vi "EditParam.vi"(10 "type":u16(ring)=2 items=["USB-CAN"=2, "USB-CAN2.0"=3], 11 "param":T1[](array[typedef]) {"ACR0" format="%x"}) -> (3 "param out":T1[](array[typedef]) {"ACR0" format="%x"})   [LabVIEW 2011]
uses:
  Param.ctl
panel:
  in  "m2":enum16{"ANY", "IDE"}(ring) caption="过滤模式:"
  in  "m1":enum16{"标准帧", "扩展帧"}(ring) caption="过滤模式:"
  in  "m0":enum16{"标准帧", "扩展帧"}(ring) caption="过滤模式组合:"
  in  "Cancel":bool
  in  "OK":bool
  in  "channel":enum16{"通道1", "通道2"}(ring) caption="选择要编辑的CAN通道号："
  in  "屏蔽码":u32=4294967295 caption="屏蔽码:" format="0x%08x"
  in  "验收码":u32=2147483648 caption="验收码:" format="0x%08x"
  in  "工作模式:":u16(ring) items=["正常工作", "自测模试（环回模式）", "仅监帧听模式", "监听所有信息模式", "关闭模式", "配置模式"]
  in  "BTR1":u8=28 caption="(HEX)" format="%02x"
  in  "BTR0":u8=1 caption="BTR0/1:" format="%02x"
  in  "br":u32(ring)=8 caption="波特率:" items=["5k bps"=1, "10k bps"=2, "20k bps"=3, "40k bps"=4, "50k bps"=5, "80k bps"=6, "100k bps"=7, "125k bps"=8, "200k bps"=9, "250k bps"=10, "400k bps"=11, "500k bps"=12, "666k bps"=13, "800k bps"=14, "1000k bps"=15, "self define"=16]
  # "CAN初始化参数"
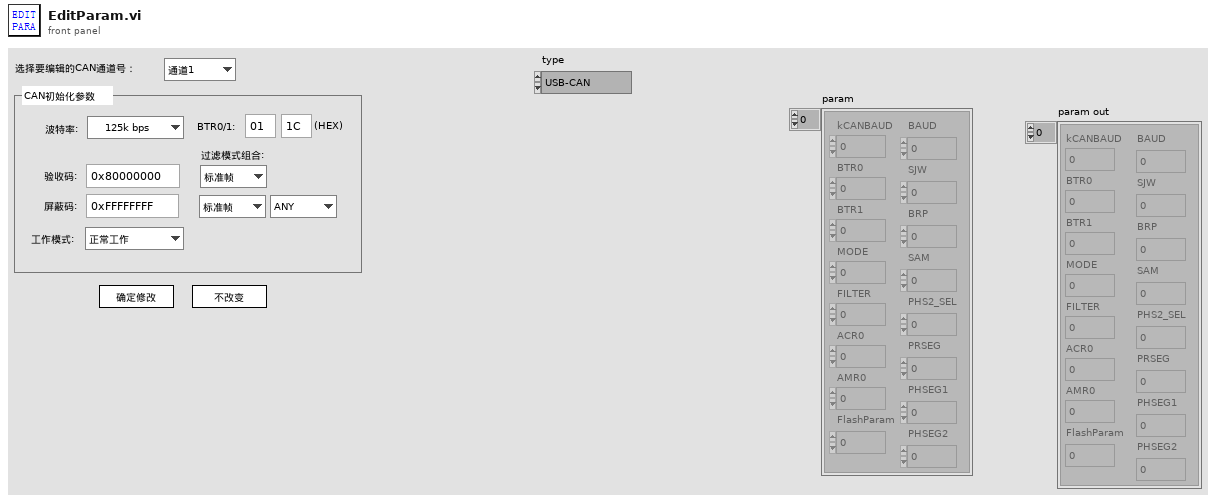
[diagram p1: front panel]
types:
  T1 = typedef "Param.ctl" = cluster{"kCANBAUD":u8, "BTR0":u8, "BTR1":u8, "MODE":u8, "FILTER":u8, "ACR0":u32, "AMR0":u32, "FlashParam":u32, "BAUD":u32, "SJW":u8, "BRP":u8, "SAM":u8, "PHS2_SEL":u8, "PRSEG":u8, "PHSEG1":u8, "PHSEG2":u8}
  T2 = enum8{"Enabled", "Disabled", "Disabled and Grayed Out"}
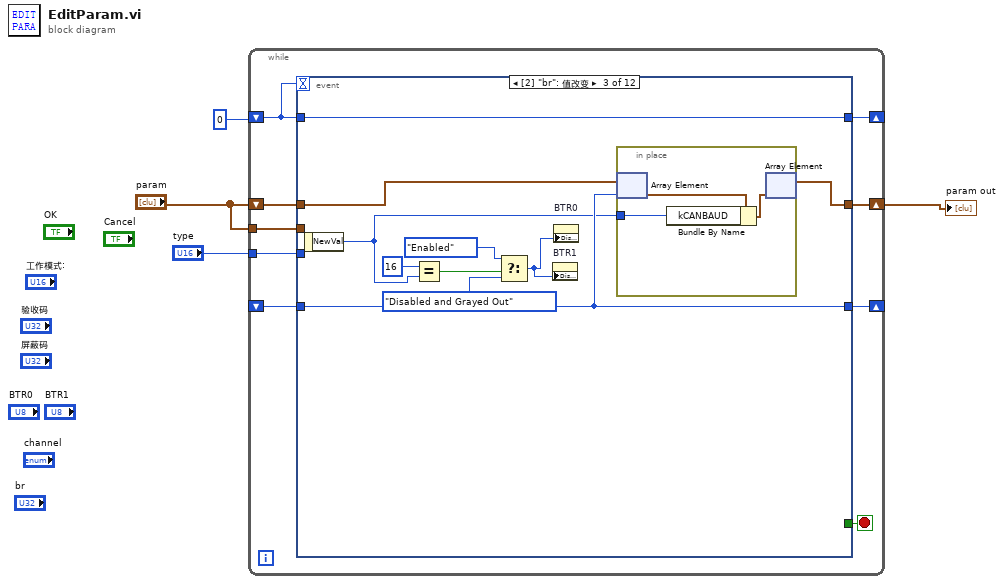
[diagram p0: block diagram]
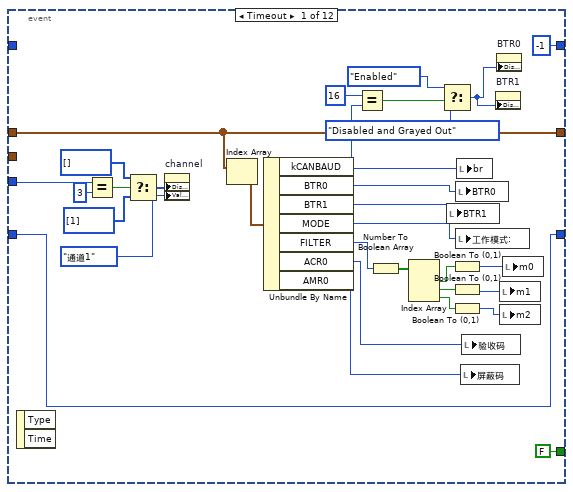
[diagram p2: hidden frame]
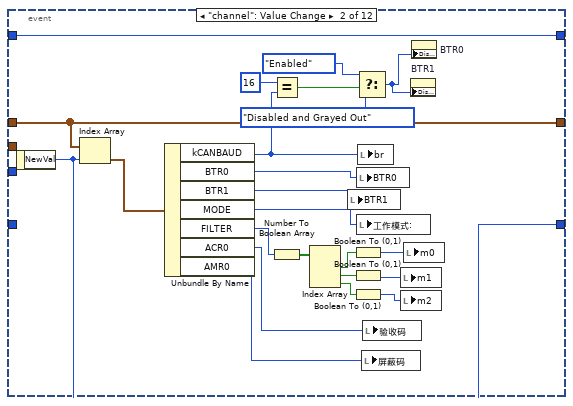
[diagram p3: hidden frame]
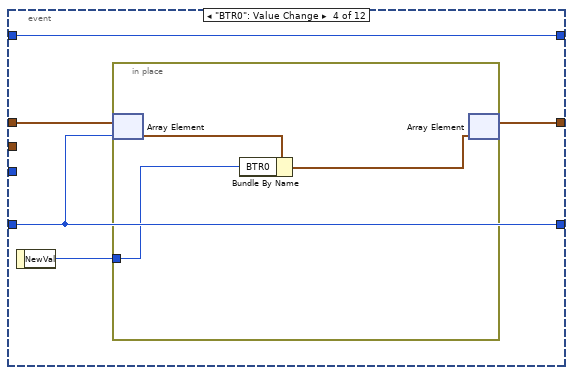
[diagram p4: hidden frame]
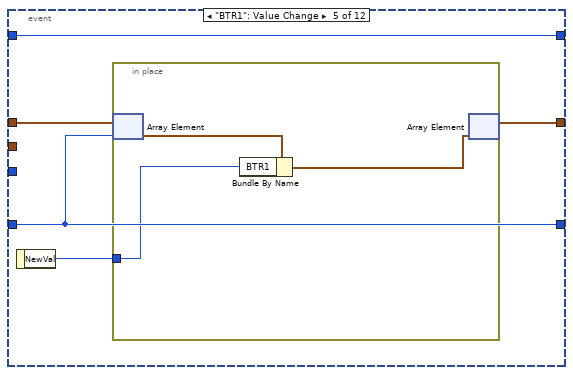
[diagram p5: hidden frame]
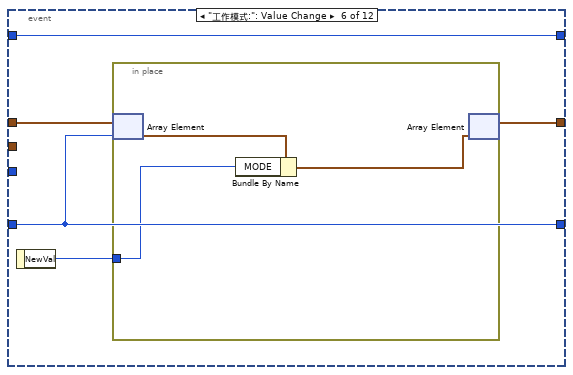
[diagram p6: hidden frame]
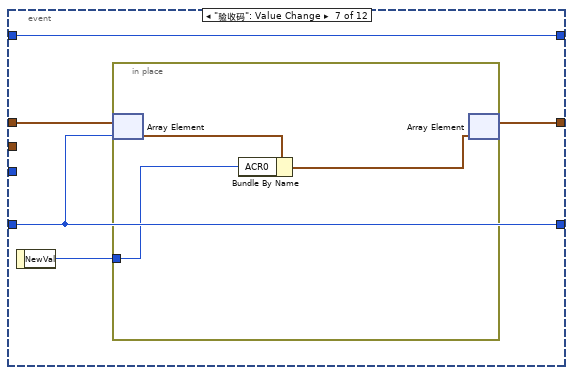
[diagram p7: hidden frame]
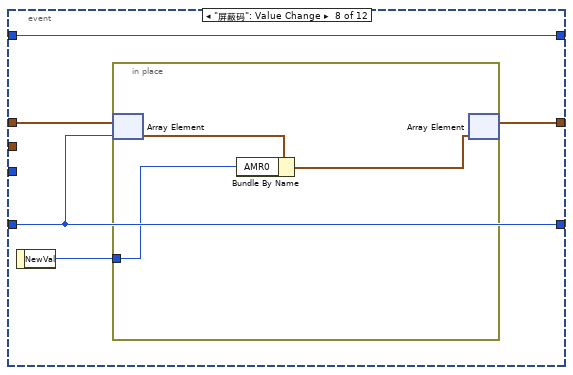
[diagram p8: hidden frame]
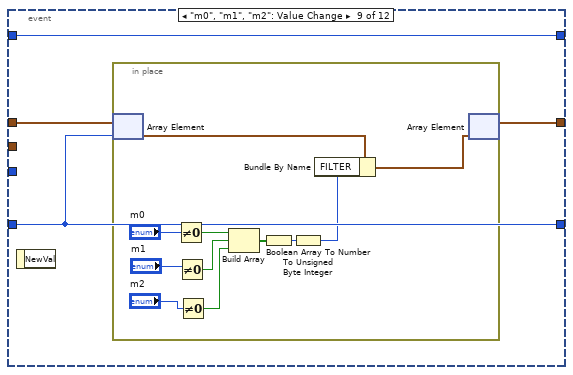
[diagram p9: hidden frame]
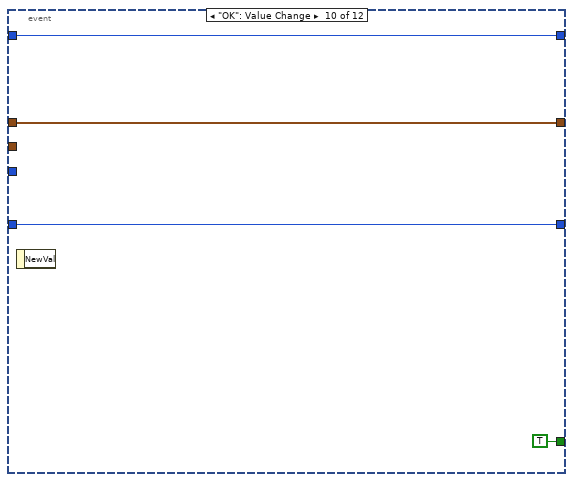
[diagram p10: hidden frame]
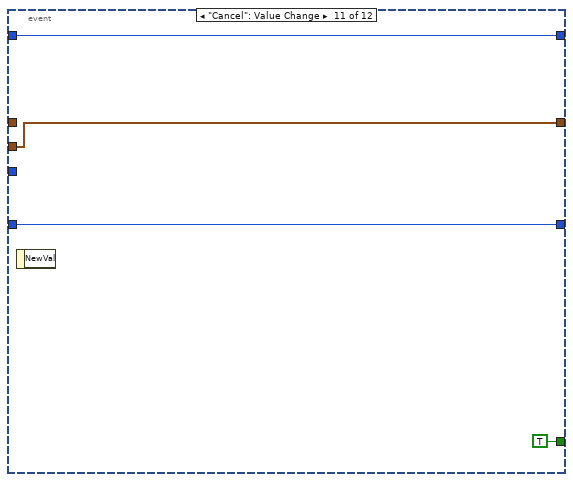
[diagram p11: hidden frame]
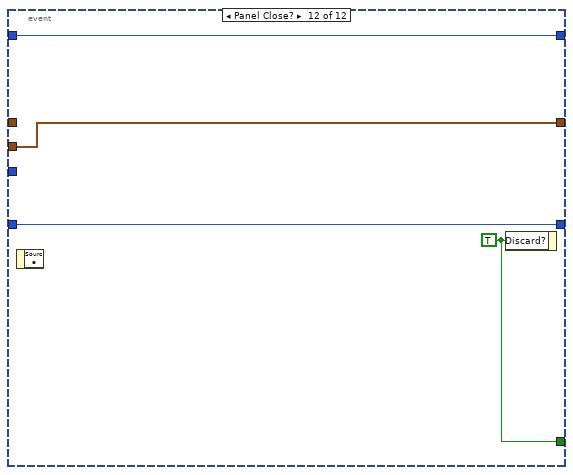
[diagram p12: hidden frame]
diagram:
  n1 = while {
    shift-right: [w11] -> w2
    shift-left: "param" -> [w12]
    shift-right: [w10] -> _
    shift-left: 0 -> [w9]
    tunnel: "type" -> [w8]
    shift-right: [w7] -> _
    shift-left: _ -> [w6]
    tunnel: "param" -> [w5]
    stop <- w13 stop-if-true
    n2 = event shown="[2] \"br\": 值改变" {
      selector: _ -> [_ _ _ _ _ _ _ _ _ _ _ _]
      dyn-events: _ -> [_ _ _ _ _ _ _ _ _ _ _ _]
      timeout: w9 -> [_ _ _ _ _ _ _ _ _ _ _ _]
      tunnel: [FALSE _ _ _ _ _ _ _ _ TRUE TRUE w145] -> w13
      tunnel: w12 -> [w35 w66 w71 w84 w92 w100 w108 w116 w123 w139 _ _]
      tunnel: [w35 w66 w69 w82 w90 w98 w106 w114 w122 w139 w140 w144] -> w11
      tunnel: [-1 w67 w77 w85 w93 w101 w109 w117 w124 w138 w143 w147] -> w10
      tunnel: w9 -> [_ w67 w77 w85 w93 w101 w109 w117 w124 w138 w143 w147]
      tunnel: w8 -> [w42 _ _ _ _ _ _ _ _ _ _ _]
      tunnel: [w14 w45 w70 w81 w89 w97 w105 w113 w121 w137 w142 w146] -> w7
      tunnel: w6 -> [w14 _ w70 w81 w89 w97 w105 w113 w121 w137 w142 w146]
      tunnel: w5 -> [_ _ _ _ _ _ _ _ _ _ w140 w144]
      event Timeout {
        n3 = event-data() -> ()  [unwired: 1 in, 2 out]
        n4 = Equal?(x=w42, y=u16 3) -> (x = y?=w40:bool)
        n5 = Select(t=i32[] [] ("禁用项[]"), s=w40, f=i32[] [1] ("禁用项[]")) -> (s? t:f=w37:i32[])
        n6 = property on="channel" class="Enum (严格)"("Disabled Items []"=w37, "Value"=enum16{"通道1", "通道2"}."通道1" ("channel")) -> ()  [unwired: 2 in, 2 out]
        n7 = Index Array(array=w35) -> (element=w34:T1)  [unwired: 1 in]
        n8 = Unbundle By Name(w34) -> ("kCANBAUD"=w20:u8, "BTR0"=w33:u8, "BTR1"=w32:u8, "MODE"=w31:u8, "FILTER"=w26:u8, "ACR0"=w22:u32, "AMR0"=w21:u32)
        n9 = Equal?(x=u8 16, y=w20) -> (x = y?=w16:bool)
        n10 = Number To Boolean Array(number=w26) -> (Boolean array=w30:bool[])
        n11 = Index Array(array=w30) -> (element #1=w29:bool, element #2=w28:bool, element #3=w27:bool)  [unwired: 3 in]
        n12 = Select(t=T2."Enabled" ("禁用"), s=w16, f=T2."Disabled and Grayed Out") -> (s? t:f=w15:T2)
        n13 = local write "BTR1"(w32) -> ()
        n14 = Boolean To (0,1)(Boolean=w29) -> (0, 1=w25:i16)
        n15 = Boolean To (0,1)(Boolean=w28) -> (0, 1=w24:i16)
        n16 = Boolean To (0,1)(Boolean=w27) -> (0, 1=w23:i16)
        n17 = local write "BTR0"(w33) -> ()
        n18 = local write "工作模式:"(w31) -> ()
        n19 = local write "br"(w20) -> ()
        n20 = local write "屏蔽码"(w21) -> ()
        n21 = local write "验收码"(w22) -> ()
        n22 = property on="BTR1" class="DigNum (严格)"("DisabledEnum"=w15) -> ()  [unwired: 2 in, 2 out]
        n23 = property on="BTR0" class="DigNum (严格)"("DisabledEnum"=w15) -> ()  [unwired: 2 in, 2 out]
        n24 = local write "m1"(w24) -> ()
        n25 = local write "m2"(w23) -> ()
        n26 = local write "m0"(w25) -> ()
      }
      event "channel": Value Change {
        n27 = event-data() -> ("NewVal"=w45:enum16{"通道1", "通道2"})  [unwired: 1 in]
        n28 = Index Array(array=w66, index=w45) -> (element=w52:T1)
        n29 = Unbundle By Name(w52) -> ("kCANBAUD"=w46:u8, "BTR0"=w65:u8, "BTR1"=w64:u8, "MODE"=w63:u8, "FILTER"=w58:u8, "ACR0"=w54:u32, "AMR0"=w53:u32)
        n30 = Equal?(x=u8 16, y=w46) -> (x = y?=w48:bool)
        n31 = Number To Boolean Array(number=w58) -> (Boolean array=w62:bool[])
        n32 = Index Array(array=w62) -> (element #1=w61:bool, element #2=w60:bool, element #3=w59:bool)  [unwired: 3 in]
        n33 = local write "BTR1"(w64) -> ()
        n34 = Boolean To (0,1)(Boolean=w61) -> (0, 1=w57:i16)
        n35 = Boolean To (0,1)(Boolean=w60) -> (0, 1=w56:i16)
        n36 = Boolean To (0,1)(Boolean=w59) -> (0, 1=w55:i16)
        n37 = Select(t=T2."Enabled" ("禁用"), s=w48, f=T2."Disabled and Grayed Out") -> (s? t:f=w47:T2)
        n38 = local write "BTR0"(w65) -> ()
        n39 = local write "工作模式:"(w63) -> ()
        n40 = local write "br"(w46) -> ()
        n41 = local write "屏蔽码"(w53) -> ()
        n42 = local write "验收码"(w54) -> ()
        n43 = local write "m1"(w56) -> ()
        n44 = local write "m2"(w55) -> ()
        n45 = local write "m0"(w57) -> ()
        n46 = property on="BTR1" class="DigNum (严格)"("DisabledEnum"=w47) -> ()  [unwired: 2 in, 2 out]
        n47 = property on="BTR0" class="DigNum (严格)"("DisabledEnum"=w47) -> ()  [unwired: 2 in, 2 out]
      }
      event "br": Value Change {
        n48 = event-data() -> ("NewVal"=w68:u32)  [unwired: 1 in]
        n49 = Equal?(x=u8 16, y=w68) -> (x = y?=w75:bool)
        n50 = Select(t=T2."Enabled" ("禁用"), s=w75, f=T2."Disabled and Grayed Out") -> (s? t:f=w74:T2)
        n51 = property on="BTR1" class="DigNum (严格)"("DisabledEnum"=w74) -> ()  [unwired: 2 in, 2 out]
        n52 = property on="BTR0" class="DigNum (严格)"("DisabledEnum"=w74) -> ()  [unwired: 2 in, 2 out]
        n53 = in-place {
          in-place-border: w68 -> [w78]
          n54 = in-place-array #1(w71, w70) -> (w80:T1)
          n55 = Bundle By Name(cluster=w80, "kCANBAUD"=w78) -> (w79:T1)
          n56 = in-place-array #1(w79) -> (w69:T1[])  [unwired: 1 out]
        }
      }
      event "BTR0": Value Change {
        n57 = event-data() -> ("NewVal"=w83:u8)  [unwired: 1 in]
        n58 = in-place {
          in-place-border: w83 -> [w87]
          n59 = in-place-array #2(w84, w81) -> (w88:T1)
          n60 = Bundle By Name(cluster=w88, "BTR0"=w87) -> (w86:T1)
          n61 = in-place-array #2(w86) -> (w82:T1[])  [unwired: 1 out]
        }
      }
      event "BTR1": Value Change {
        n62 = event-data() -> ("NewVal"=w91:u8)  [unwired: 1 in]
        n63 = in-place {
          in-place-border: w91 -> [w95]
          n64 = in-place-array #3(w92, w89) -> (w96:T1)
          n65 = Bundle By Name(cluster=w96, "BTR1"=w95) -> (w94:T1)
          n66 = in-place-array #3(w94) -> (w90:T1[])  [unwired: 1 out]
        }
      }
      event "工作模式:": Value Change {
        n67 = event-data() -> ("NewVal"=w99:u16)  [unwired: 1 in]
        n68 = in-place {
          in-place-border: w99 -> [w103]
          n69 = in-place-array #4(w100, w97) -> (w104:T1)
          n70 = Bundle By Name(cluster=w104, "MODE"=w103) -> (w102:T1)
          n71 = in-place-array #4(w102) -> (w98:T1[])  [unwired: 1 out]
        }
      }
      event "验收码": Value Change {
        n72 = event-data() -> ("NewVal"=w107:u32)  [unwired: 1 in]
        n73 = in-place {
          in-place-border: w107 -> [w111]
          n74 = in-place-array #5(w108, w105) -> (w112:T1)
          n75 = Bundle By Name(cluster=w112, "ACR0"=w111) -> (w110:T1)
          n76 = in-place-array #5(w110) -> (w106:T1[])  [unwired: 1 out]
        }
      }
      event "屏蔽码": Value Change {
        n77 = event-data() -> ("NewVal"=w115:u32)  [unwired: 1 in]
        n78 = in-place {
          in-place-border: w115 -> [w119]
          n79 = in-place-array #6(w116, w113) -> (w120:T1)
          n80 = Bundle By Name(cluster=w120, "AMR0"=w119) -> (w118:T1)
          n81 = in-place-array #6(w118) -> (w114:T1[])  [unwired: 1 out]
        }
      }
      event "m0", "m1", "m2": Value Change {
        n82 = event-data() -> ()  [unwired: 1 in, 1 out]
        n83 = in-place {
          n84 = in-place-array #7(w123, w121) -> (w135:T1)
          n85 = Not Equal To 0?(x="m0") -> (x != 0?=w133:bool)
          n86 = Not Equal To 0?(x="m1") -> (x != 0?=w132:bool)
          n87 = Not Equal To 0?(x="m2") -> (x != 0?=w131:bool)
          n88 = Build Array(w133, w132, w131) -> (w130:bool[])
          n89 = Boolean Array To Number(Boolean array=w130) -> (number=w129:u32)
          n90 = To Unsigned Byte Integer(number=w129) -> (unsigned 8bit integer=w125:u8)
          n91 = Bundle By Name(cluster=w135, "FILTER"=w125) -> (w134:T1)
          n92 = in-place-array #7(w134) -> (w122:T1[])  [unwired: 1 out]
        }
      }
      event "OK": Value Change {
        n93 = event-data() -> ()  [unwired: 1 in, 1 out]
      }
      event "Cancel": Value Change {
        n94 = event-data() -> ()  [unwired: 1 in, 1 out]
      }
      event Panel Close? {
        w145 = TRUE ("放弃？")
        n95 = event-data() -> ()  [unwired: 1 in, 1 out]
        n96 = event-data("Discard?"=w145) -> ()  [unwired: 1 in, 1 out]
      }
    }
  }
  "param out" <- w2
